vi "niRFUtil MEAS Compensate IQ Imbalances.vi"(8 "Compensate?":bool, 9 "Input":T1 {"y" format="%.2f"; "dx" format="%^.2e"; "x0" format="%^.2e"}, 11 "Imbalance Matrix":T3) -> (3 "Waveform Out":T1 {"y" format="%.2f"; "dx" format="%^.2e"; "x0" format="%^.2e"})   [LabVIEW 2015, in "niRFUtil.lvlib"]
uses:
  niRFUtil.lvlib
  <vilib>/Analysis/Matrix/Datatypes/RealMatrix.ctl
  Includes/niRFUtil INC Complex Waveform.ctl
  Includes/niRFUtil INC Complex Array.ctl
  <vilib>/Analysis/baseanly.llb/Real A x B.vi
  <vilib>/Analysis/baseanly.llb/Real Inverse Matrix.vi
  <vilib>/Analysis/NI_AALBase.lvlib
  <vilib>/Analysis/Matrix/NI_Matrix.lvlib
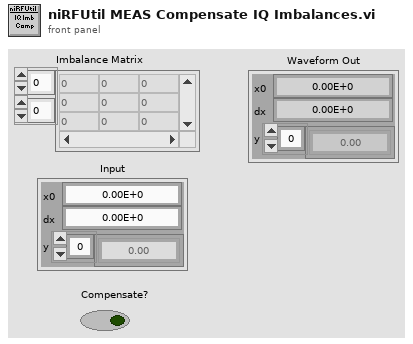
[diagram p1: front panel]
types:
  T1 = typedef "niRFUtil.lvlib/niRFUtil INC Complex Waveform.ctl" = cluster{"x0":dbl, "dx":dbl, "y":T2}
  T2 = typedef "niRFUtil.lvlib/niRFUtil INC Complex Array.ctl" = csg[]
  T3 = typedef "NI_Matrix.lvlib/RealMatrix.ctl" = dbl[][]
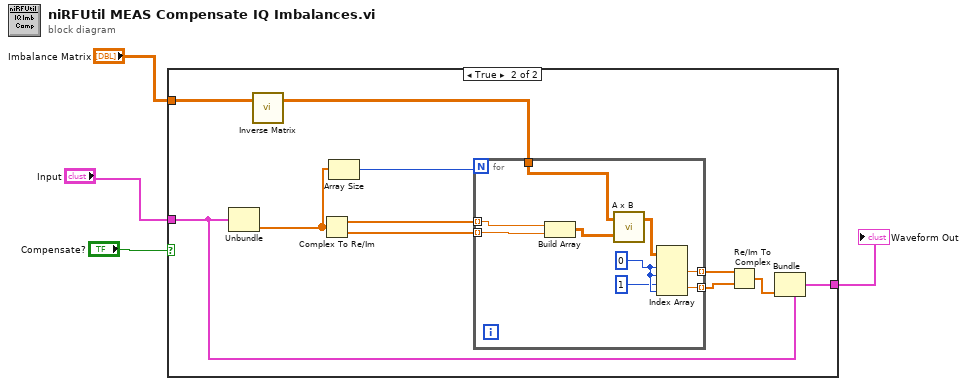
[diagram p0: block diagram]
diagram:
  n1 = case shown="True" "Compensate?" {
    tunnel: "Imbalance Matrix" -> [_ w16]
    tunnel: "Input" -> [w5 w6]
    tunnel: [w5 w7] -> w3
    frame False {
    }
    frame True {
      n2 = Unbundle(w6) -> ("y"=w8:T2)  [unwired: 2 out]
      n3 = call-poly <vilib>:"Inverse Matrix.vi"("Input Matrix"=w16) -> ("Inverse Matrix"=w12:T3)  [unwired: 1 in, 1 out]
      n4 = Complex To Re/Im(x + iy=w8) -> (x=w14:sgl[], y=w13:sgl[])
      n5 = Array Size(array=w8) -> (size(s)=w15:i32)
      n6 = for {
        N: w15 -> [_]
        tunnel: w14 -> [w25] mode=indexing
        tunnel: w13 -> [w24] mode=indexing
        tunnel: w12 -> [w19]
        tunnel: [w22] -> w11 mode=indexing
        tunnel: [w21] -> w10 mode=indexing
        w18 = 0 ("index (row)")
        n7 = Build Array(w25, w24) -> (w20:T3)
        n8 = call-poly <vilib>:"A x B.vi"("B"=w20, "A"=w19) -> ("A x B"=w23:T3)  [unwired: 1 out]
        n9 = Index Array(array=w23, index (row) #1=w18, index (col) #1=w18, index (row) #2=1 ("index (row)"), index (col) #2=w18) -> (element #1=w22:dbl, element #2=w21:dbl)
      }
      n10 = Re/Im To Complex(1:w10, 2:w11) -> (0:w9:cdb[])
      n11 = Bundle(cluster=w6, "y"=w9) -> (w7:T1)  [unwired: 2 in]
    }
  }
  "Waveform Out" <- w3
